vi "Close.vi"(8 "error in (no error)":errorcluster, 11 "Function in":refnum<class "Function.lvclass">) -> (0 "error out":errorcluster, 3 "Function out":refnum<class "Function.lvclass">)   [LabVIEW 2016, in "Function Actor.lvlib" / "Function.lvclass"]
uses:
  <userlib>/Common Components/Function Actor/Function.lvclass
  <userlib>/Common Components/Function Actor/Function.lvclass/Function.ctl
  <vilib>/MediaMongrels Ltd/WebSockets/WebSockets/WebSockets.lvlib
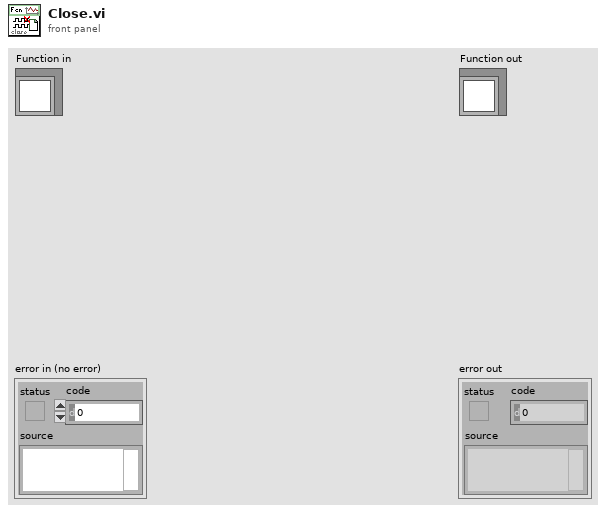
[diagram p1: front panel]
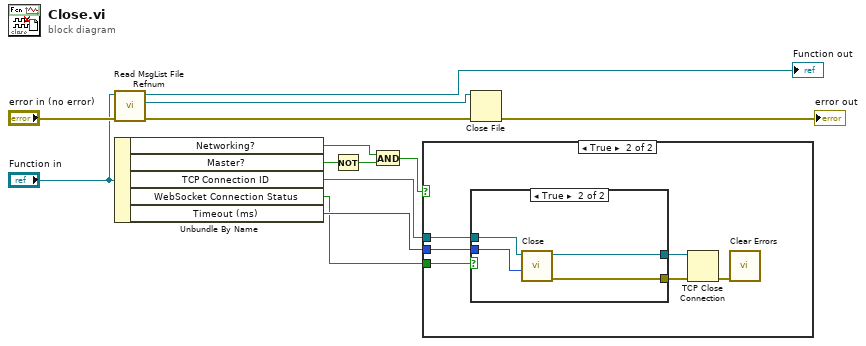
[diagram p0: block diagram]
diagram:
  n1 = call <userlib>:"Read MsgList File Refnum.vi"("error in (no error)"="error in (no error)", "Function in"="Function in") -> ("error out"=w10:errorcluster, "Cmd List File Refnum"=w11:refnum<file>, "Function out"=→"Function out":refnum<class "Function.lvclass">)  [unwired: 7 in]
  n2 = Unbundle By Name("Function in") -> ("Networking?"=w7:bool, "Master?"=w8:bool, "TCP Connection ID"=w3:refnum<k5>, "WebSocket Connection Status"=w1:bool, "Timeout (ms)"=w2:i32)
  n3 = Not(x=w8) -> (.not. x?=w6:bool)
  n4 = And(x=w7, y=w6) -> (x .and. y?=w4:bool)
  n5 = case shown="True" w4 {
    tunnel: w3 -> [_ w18]
    tunnel: w2 -> [_ w17]
    tunnel: w1 -> [_ w15]
    frame False {
    }
    frame True {
      n6 = case shown="True" w15 {
        tunnel: w18 -> [w20 w24]
        tunnel: w17 -> [_ w23]
        tunnel: [_ w22] -> w16
        tunnel: [w20 w21] -> w14
        frame False {
        }
        frame True {
          n7 = call <vilib>:"Close.vi"("timeout ms (5000)"=w23, "WebSocket Connection in"=w24) -> ("error out"=w22:errorcluster, "WebSocket Connection in"=w21:refnum<k5>)  [unwired: 8 in]
        }
      }
      n8 = TCP Close Connection(connection ID=w14, error in (no error)=w16) -> (error out=w19:errorcluster)  [unwired: 1 in, 1 out]
      n9 = call <vilib>:"Clear Errors.vi"("error in (no error)"=w19) -> ()  [unwired: 5 in, 2 out]
    }
  }
  n10 = Close File(refnum=w11, error in=w10) -> (error out=→"error out":errorcluster)  [unwired: 1 out]
